vi "2 dof forward.vi"() -> ()   [LabVIEW 2021]
panel:
  out "Coordinates":cluster{"x":dbl, "y":dbl, "y 2":dbl}
  in  "Parameters of 2 DOF":T1={"Theta Motor 1"=0.0, "Theta Motor 2"=0.0, "l1"=230.59, "l2"=112.96} caption="Parameters of Delta Robot"
  # "Definitions about the Inputs of Forward Kinematics :"
  # "Theta Motor 1 , Theta Motor 2 represents the angles of two smart motors of 2 DOF."
  # "l1 and l2 respresents links length."
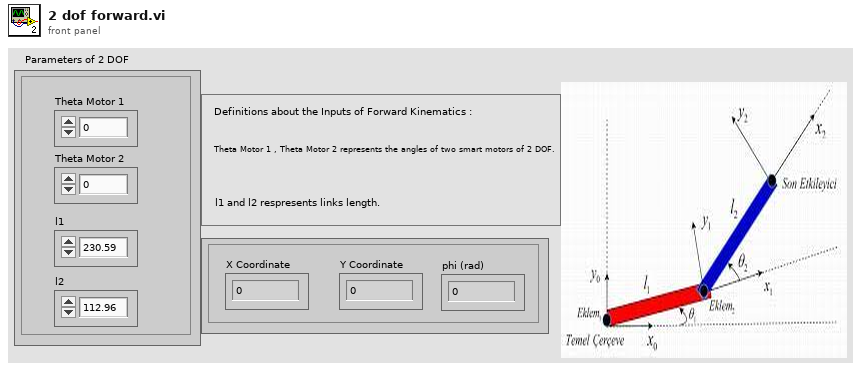
[diagram p1: front panel]
types:
  T1 = cluster{"Theta Motor 1":dbl, "Theta Motor 2":dbl, "l1":dbl, "l2":dbl}
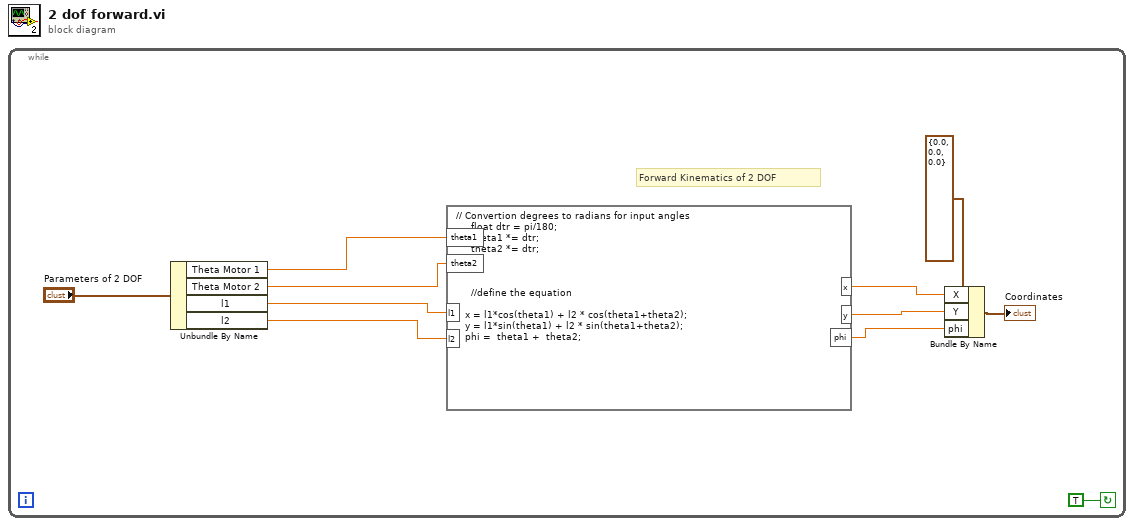
[diagram p0: block diagram]
diagram:
  n1 = while {
    stop <- TRUE continue-if-true
    # "Forward Kinematics of 2 DOF"
    n2 = Unbundle By Name "Unbundle By Name"("Parameters of 2 DOF") -> ("Theta Motor 1"=w7:dbl, "Theta Motor 2"=w9:dbl, "l1"=w11:dbl, "l2"=w10:dbl)
    n3 = formula code="// Convertion degrees to radians for input angles\n     float dtr = pi/180;\n     theta1 *= dtr;\n     theta2 *= dtr;\n     \n     \n  \n     //define the equation\n\n   x = l1*cos(theta1) + l2 * cos(theta1+theta2);\n   y = l1*sin(theta1) + l2 * sin(theta1+theta2);\n   phi =  theta1 +  theta2;"("theta1"=w7, "theta2"=w9, "l1"=w11, "l2"=w10) -> ("x"=w6:dbl, "y"=w4:dbl, "phi"=w1:dbl)
    n4 = Bundle By Name(cluster=cluster{"X":dbl, "Y":dbl, "phi":dbl} {"X"=0.0, "Y"=0.0, "phi"=0.0}, "X"=w6, "Y"=w4, "phi"=w1) -> (→"Coordinates":cluster{"X":dbl, "Y":dbl, "phi":dbl})
  }
